vi "Day 5.2.vi"(11 "input":string[](array[string])) -> (3 "ouptut part 2":u64)   [LabVIEW 2021]
uses:
  <vilib>/regexp/Match Regular Expression.xnode
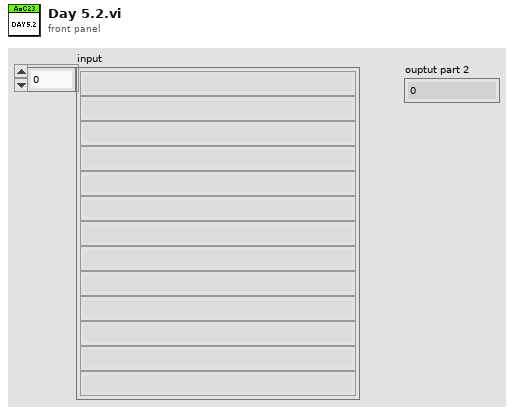
[diagram p1: front panel]
types:
  T1 = cluster{"From":string, "To":string, "dest-source-range":u64[][]}
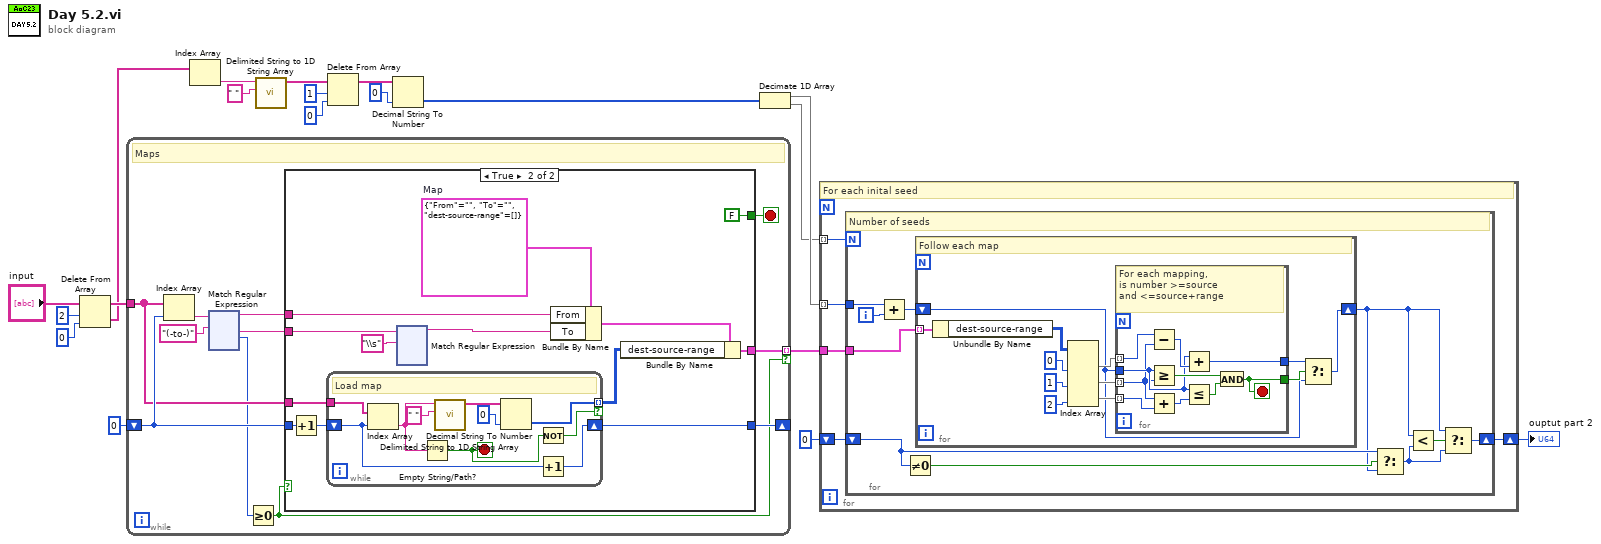
[diagram p0: block diagram]
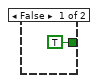
[diagram p2: hidden frame]
diagram:
  n1 = Delete From Array(array="input", length=2, index=0) -> (deleted portion=w16:string[], array with subset deleted=w17:string[])
  n2 = while {
    tunnel: w17 -> [w25]
    shift-right: [w24] -> _
    shift-left: 0 -> [w26]
    tunnel: [w23] -> w3 mode=indexing if=w21
    stop <- w20 stop-if-true
    # "Maps"
    n3 = Index Array(array=w25, index=w26) -> (element=w27:string)
    n4 = xnode "Match Regular Expression"("input string"=w27, "regular expression"="(-to-)") -> ("before match"=w29:string, "after match"=w28:string, "offset past match"=w22:i32)  [unwired: 4 in, 2 out]
    n5 = Greater Or Equal To 0?(x=w22) -> (x >= 0?=w21:bool)
    n6 = case shown="True" w21 {
      tunnel: w29 -> [_ w43]
      tunnel: w28 -> [_ w42]
      tunnel: w26 -> [_ w39]
      tunnel: w25 -> [_ w37]
      tunnel: [_ w34] -> w24
      tunnel: [_ w33] -> w23
      tunnel: [TRUE FALSE] -> w20
      frame False {
      }
      frame True {
        w44 = T1 {"From"="", "To"="", "dest-source-range"=[]}  # Map
        n7 = Increment(x=w39) -> (x+1=w38:i32)
        n8 = while {
          shift-right: [w46] -> w34
          shift-left: w38 -> [w47]
          tunnel: w37 -> [w54]
          tunnel: [w50] -> w35 mode=indexing if=w48
          stop <- w49 stop-if-true
          # "Load map"
          n9 = Index Array(array=w54, index=w47) -> (element=w52:string)
          n10 = Empty String/Path?(string/path=w52) -> (empty?=w49:bool)
          n11 = call <vilib>:"Delimited String to 1D String Array.vi"("delimiter"=" ", "delimited string"=w52) -> ("string array"=w51:string[])  [unwired: 9 in]
          n12 = Decimal String To Number(string=w51, default (0L)=u64 0 ("default (0 I32)")) -> (number=w50:u64[])  [unwired: 1 in, 1 out]
          n13 = Not(x=w49) -> (.not. x?=w48:bool)
          n14 = Increment(x=w47) -> (x+1=w46:i32)
        }
        n15 = xnode "Match Regular Expression"("input string"=w42, "regular expression"="\\s") -> ("before match"=w40:string)  [unwired: 4 in, 4 out]
        n16 = Bundle By Name(cluster=w44, "From"=w43, "To"=w40) -> (w36:T1)
        n17 = Bundle By Name(cluster=w36, "dest-source-range"=w35) -> (w33:T1)
      }
    }
  }
  n18 = Index Array(array=w16) -> (element=w15:string)  [unwired: 1 in]
  n19 = call <vilib>:"Delimited String to 1D String Array.vi"("delimiter"=" ", "delimited string"=w15) -> ("string array"=w13:string[])  [unwired: 9 in]
  n20 = Delete From Array(array=w13, length=1, index=0) -> (array with subset deleted=w10:string[])  [unwired: 1 out]
  n21 = Decimal String To Number(string=w10, default (0L)=u64 0 ("default (0 I32)")) -> (number=w7:u64[])  [unwired: 1 in, 1 out]
  n22 = Decimate 1D Array(w7) -> (w6:u64[], w5:u64[])
  n23 = for {
    tunnel: w6 -> [w292] mode=indexing
    tunnel: w5 -> [w293] mode=indexing
    shift-right: [w289] -> w2
    shift-left: u64 0 -> [w290]
    tunnel: w3 -> [w291]
    # "For each inital seed"
    n24 = for {
      N: w293 -> [_]
      tunnel: w292 -> [w302]
      tunnel: w291 -> [w301]
      shift-right: [w295] -> w289
      shift-left: w290 -> [w297]
      i -> [w303]
      # "Number of seeds"
      n25 = Add(x=w302, y=w303) -> (x+y=w300:u64)
      n26 = Not Equal To 0?(x=w297) -> (x != 0?=w298:bool)
      n27 = for {
        tunnel: w301 -> [w315] mode=indexing
        shift-right: [w304] -> w296
        shift-left: w300 -> [w305]
        # "Follow each map"
        n28 = Unbundle By Name(w315) -> ("dest-source-range"=w314:u64[][])
        n29 = Index Array(array=w314, index (col) #1=0 ("disabled index (col)"), index (col) #2=1 ("index (col)"), index (col) #3=2 ("index (col)")) -> (element #1=w310:u64[], element #2=w309:u64[], element #3=w308:u64[])  [unwired: 3 in]
        n30 = for {
          tunnel: w310 -> [w318] mode=indexing
          tunnel: w309 -> [w316] mode=indexing
          tunnel: w308 -> [w325] mode=indexing
          tunnel: w305 -> [w317]
          tunnel: [w320] -> w306
          tunnel: [w319] -> w307
          stop <- w319 stop-if-true
          # "For each mapping,\nis number >=source\nand <=source+range"
          n31 = Subtract(x=w318, y=w316) -> (x-y=w321:u64)
          n32 = Greater Or Equal?(x=w317, y=w316) -> (x >= y?=w323:bool)
          n33 = Add(x=w316, y=w325) -> (x+y=w324:u64)
          n34 = Add(x=w317, y=w321) -> (x+y=w320:u64)
          n35 = Less Or Equal?(x=w317, y=w324) -> (x <= y?=w322:bool)
          n36 = And(x=w323, y=w322) -> (x .and. y?=w319:bool)
        }
        n37 = Select(t=w306, s=w307, f=w305) -> (s? t:f=w304:u64)
      }
      n38 = Select(t=w297, s=w298, f=w296) -> (s? t:f=w294:u64)
      n39 = Less?(x=w296, y=w294) -> (x < y?=w299:bool)
      n40 = Select(t=w296, s=w299, f=w294) -> (s? t:f=w295:u64)
    }
  }
  "ouptut part 2" <- w2
